vi "PacketID_generator.vi"() -> (3 "PacketId":u16)   [LabVIEW 2018, in "MQTT_Functions.lvlib"]
uses:
  MQTT_Functions.lvlib
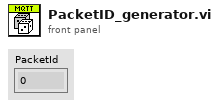
[diagram p1: front panel]
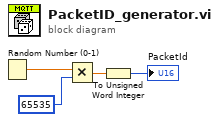
[diagram p0: block diagram]
diagram:
  n1 = Random Number (0-1)() -> (number: 0 to 1=w4:dbl)
  n2 = Multiply(x=w4, y=u16 65535) -> (x*y=w2:dbl)
  n3 = To Unsigned Word Integer(number=w2) -> (unsigned 16bit integer=→"PacketId":u16)
